vi "MGCC_DataLog.vi"(0 "Start 2":bool=TRUE, 2 "Start":bool=TRUE) -> ()   [LabVIEW 2016]
uses:
  <vilib>/Utility/file.llb/Write Delimited Spreadsheet (DBL).vi
panel:
  in  "Start 3":bool=TRUE
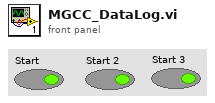
[diagram p1: front panel]
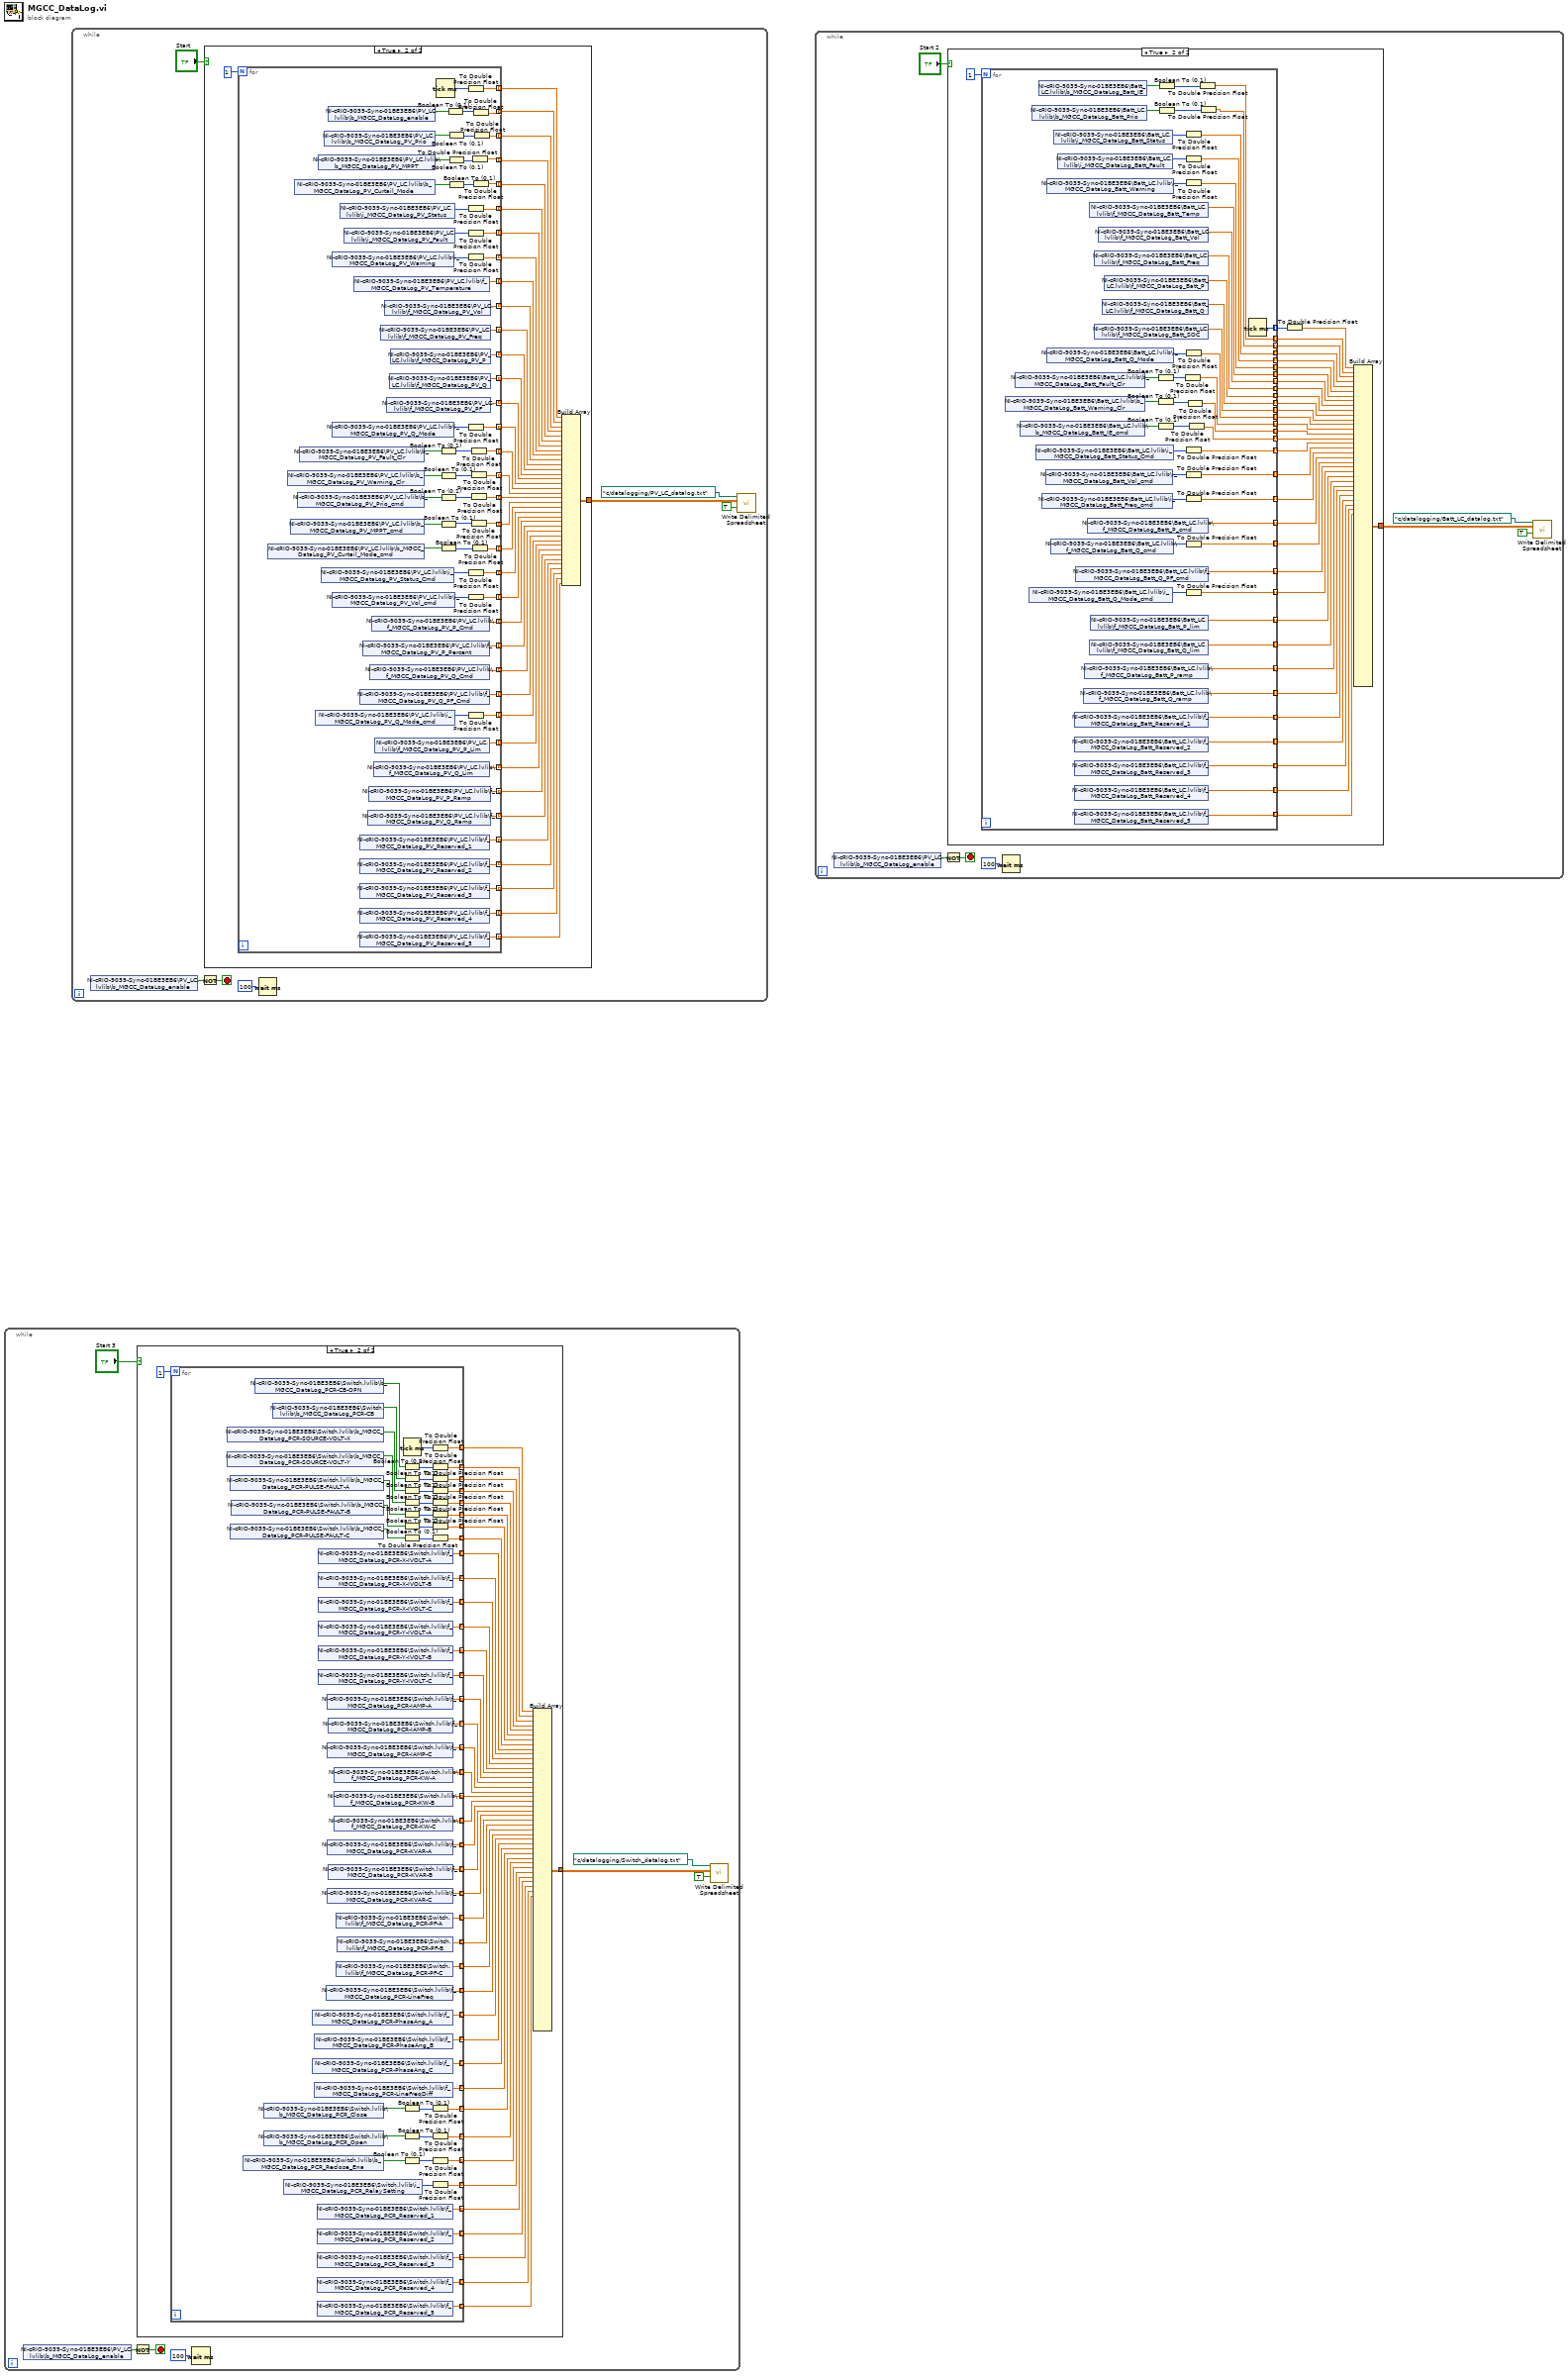
[diagram p0: block diagram]
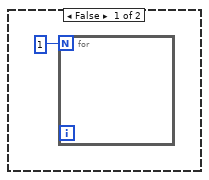
[diagram p2: hidden frame]
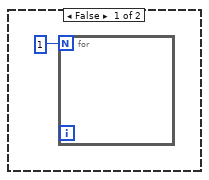
[diagram p3: hidden frame]
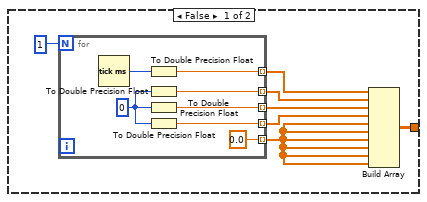
[diagram p4: hidden frame]
diagram:
  n1 = while {
    stop <- w2 stop-if-true
    n2 = shared-variable "NI-cRIO-9039-Sync-01BE3EB6\\PV_LC.lvlib\\b_MGCC_DataLog_enable"() -> (w3:bool)  [unwired: 1 in, 1 out]
    n3 = Not(x=w3) -> (.not. x?=w2:bool)
    n4 = case shown="True" "Start 3" {
      tunnel: [_ w49] -> w7
      frame False {
        n5 = for {
          N: 1 -> [_]
        }
      }
      frame True {
        n6 = for {
          N: 1 -> [_]
          tunnel: [w104] -> w48 mode=indexing
          tunnel: [w101] -> w47 mode=indexing
          tunnel: [w102] -> w46 mode=indexing
          tunnel: [w94] -> w45 mode=indexing
          tunnel: [w93] -> w44 mode=indexing
          tunnel: [w92] -> w43 mode=indexing
          tunnel: [w91] -> w42 mode=indexing
          tunnel: [w90] -> w41 mode=indexing
          tunnel: [w89] -> w40 mode=indexing
          tunnel: [w88] -> w39 mode=indexing
          tunnel: [w87] -> w38 mode=indexing
          tunnel: [w86] -> w37 mode=indexing
          tunnel: [w85] -> w36 mode=indexing
          tunnel: [w84] -> w35 mode=indexing
          tunnel: [w83] -> w34 mode=indexing
          tunnel: [w82] -> w33 mode=indexing
          tunnel: [w81] -> w32 mode=indexing
          tunnel: [w80] -> w31 mode=indexing
          tunnel: [w79] -> w30 mode=indexing
          tunnel: [w78] -> w29 mode=indexing
          tunnel: [w77] -> w28 mode=indexing
          tunnel: [w76] -> w27 mode=indexing
          tunnel: [w75] -> w26 mode=indexing
          tunnel: [w74] -> w25 mode=indexing
          tunnel: [w73] -> w24 mode=indexing
          tunnel: [w72] -> w23 mode=indexing
          tunnel: [w71] -> w22 mode=indexing
          tunnel: [w70] -> w21 mode=indexing
          tunnel: [w69] -> w20 mode=indexing
          tunnel: [w68] -> w19 mode=indexing
          tunnel: [w67] -> w18 mode=indexing
          tunnel: [w59] -> w17 mode=indexing
          tunnel: [w58] -> w16 mode=indexing
          tunnel: [w57] -> w15 mode=indexing
          tunnel: [w56] -> w14 mode=indexing
          tunnel: [w55] -> w13 mode=indexing
          tunnel: [w54] -> w12 mode=indexing
          tunnel: [w53] -> w11 mode=indexing
          tunnel: [w52] -> w10 mode=indexing
          tunnel: [w51] -> w9 mode=indexing
          n7 = shared-variable "NI-cRIO-9039-Sync-01BE3EB6\\Switch.lvlib\\b_MGCC_DataLog_PCR-SOURCE-VOLT-X"() -> (w110:bool)  [unwired: 1 in, 1 out]
          n8 = shared-variable "NI-cRIO-9039-Sync-01BE3EB6\\Switch.lvlib\\b_MGCC_DataLog_PCR-SOURCE-VOLT-Y"() -> (w109:bool)  [unwired: 1 in, 1 out]
          n9 = shared-variable "NI-cRIO-9039-Sync-01BE3EB6\\Switch.lvlib\\b_MGCC_DataLog_PCR-PULSE-FAULT-A"() -> (w108:bool)  [unwired: 1 in, 1 out]
          n10 = shared-variable "NI-cRIO-9039-Sync-01BE3EB6\\Switch.lvlib\\b_MGCC_DataLog_PCR-PULSE-FAULT-C"() -> (w106:bool)  [unwired: 1 in, 1 out]
          n11 = shared-variable "NI-cRIO-9039-Sync-01BE3EB6\\Switch.lvlib\\b_MGCC_DataLog_PCR-PULSE-FAULT-B"() -> (w107:bool)  [unwired: 1 in, 1 out]
          n12 = shared-variable "NI-cRIO-9039-Sync-01BE3EB6\\Switch.lvlib\\b_MGCC_DataLog_PCR_Reclose_Ena"() -> (w62:bool)  [unwired: 1 in, 1 out]
          n13 = shared-variable "NI-cRIO-9039-Sync-01BE3EB6\\Switch.lvlib\\b_MGCC_DataLog_PCR-CB-OPN"() -> (w112:bool)  [unwired: 1 in, 1 out]
          n14 = shared-variable "NI-cRIO-9039-Sync-01BE3EB6\\Switch.lvlib\\b_MGCC_DataLog_PCR_Close"() -> (w66:bool)  [unwired: 1 in, 1 out]
          n15 = shared-variable "NI-cRIO-9039-Sync-01BE3EB6\\Switch.lvlib\\b_MGCC_DataLog_PCR_Open"() -> (w64:bool)  [unwired: 1 in, 1 out]
          n16 = shared-variable "NI-cRIO-9039-Sync-01BE3EB6\\Switch.lvlib\\b_MGCC_DataLog_PCR-CB"() -> (w111:bool)  [unwired: 1 in, 1 out]
          n17 = shared-variable "NI-cRIO-9039-Sync-01BE3EB6\\Switch.lvlib\\i_MGCC_DataLog_PCR_RelaySetting"() -> (w60:i16)  [unwired: 1 in, 1 out]
          n18 = shared-variable "NI-cRIO-9039-Sync-01BE3EB6\\Switch.lvlib\\f_MGCC_DataLog_PCR-PhaseAng_A"() -> (w70:dbl)  [unwired: 1 in, 1 out]
          n19 = shared-variable "NI-cRIO-9039-Sync-01BE3EB6\\Switch.lvlib\\f_MGCC_DataLog_PCR-PhaseAng_C"() -> (w67:dbl)  [unwired: 1 in, 1 out]
          n20 = shared-variable "NI-cRIO-9039-Sync-01BE3EB6\\Switch.lvlib\\f_MGCC_DataLog_PCR-PhaseAng_B"() -> (w69:dbl)  [unwired: 1 in, 1 out]
          n21 = shared-variable "NI-cRIO-9039-Sync-01BE3EB6\\Switch.lvlib\\f_MGCC_DataLog_PCR-LineFreqDiff"() -> (w68:dbl)  [unwired: 1 in, 1 out]
          n22 = shared-variable "NI-cRIO-9039-Sync-01BE3EB6\\Switch.lvlib\\f_MGCC_DataLog_PCR_Reserved_1"() -> (w55:dbl)  [unwired: 1 in, 1 out]
          n23 = shared-variable "NI-cRIO-9039-Sync-01BE3EB6\\Switch.lvlib\\f_MGCC_DataLog_PCR_Reserved_2"() -> (w54:dbl)  [unwired: 1 in, 1 out]
          n24 = shared-variable "NI-cRIO-9039-Sync-01BE3EB6\\Switch.lvlib\\f_MGCC_DataLog_PCR_Reserved_3"() -> (w53:dbl)  [unwired: 1 in, 1 out]
          n25 = shared-variable "NI-cRIO-9039-Sync-01BE3EB6\\Switch.lvlib\\f_MGCC_DataLog_PCR_Reserved_4"() -> (w51:dbl)  [unwired: 1 in, 1 out]
          n26 = shared-variable "NI-cRIO-9039-Sync-01BE3EB6\\Switch.lvlib\\f_MGCC_DataLog_PCR_Reserved_5"() -> (w52:dbl)  [unwired: 1 in, 1 out]
          n27 = shared-variable "NI-cRIO-9039-Sync-01BE3EB6\\Switch.lvlib\\f_MGCC_DataLog_PCR-X-IVOLT-A"() -> (w89:dbl)  [unwired: 1 in, 1 out]
          n28 = shared-variable "NI-cRIO-9039-Sync-01BE3EB6\\Switch.lvlib\\f_MGCC_DataLog_PCR-X-IVOLT-B"() -> (w88:dbl)  [unwired: 1 in, 1 out]
          n29 = shared-variable "NI-cRIO-9039-Sync-01BE3EB6\\Switch.lvlib\\f_MGCC_DataLog_PCR-X-IVOLT-C"() -> (w87:dbl)  [unwired: 1 in, 1 out]
          n30 = shared-variable "NI-cRIO-9039-Sync-01BE3EB6\\Switch.lvlib\\f_MGCC_DataLog_PCR-Y-IVOLT-A"() -> (w86:dbl)  [unwired: 1 in, 1 out]
          n31 = shared-variable "NI-cRIO-9039-Sync-01BE3EB6\\Switch.lvlib\\f_MGCC_DataLog_PCR-Y-IVOLT-B"() -> (w85:dbl)  [unwired: 1 in, 1 out]
          n32 = shared-variable "NI-cRIO-9039-Sync-01BE3EB6\\Switch.lvlib\\f_MGCC_DataLog_PCR-Y-IVOLT-C"() -> (w84:dbl)  [unwired: 1 in, 1 out]
          n33 = shared-variable "NI-cRIO-9039-Sync-01BE3EB6\\Switch.lvlib\\f_MGCC_DataLog_PCR-LineFreq"() -> (w71:dbl)  [unwired: 1 in, 1 out]
          n34 = shared-variable "NI-cRIO-9039-Sync-01BE3EB6\\Switch.lvlib\\f_MGCC_DataLog_PCR-IAMP-A"() -> (w83:dbl)  [unwired: 1 in, 1 out]
          n35 = shared-variable "NI-cRIO-9039-Sync-01BE3EB6\\Switch.lvlib\\f_MGCC_DataLog_PCR-IAMP-C"() -> (w81:dbl)  [unwired: 1 in, 1 out]
          n36 = shared-variable "NI-cRIO-9039-Sync-01BE3EB6\\Switch.lvlib\\f_MGCC_DataLog_PCR-KVAR-A"() -> (w77:dbl)  [unwired: 1 in, 1 out]
          n37 = shared-variable "NI-cRIO-9039-Sync-01BE3EB6\\Switch.lvlib\\f_MGCC_DataLog_PCR-KVAR-C"() -> (w75:dbl)  [unwired: 1 in, 1 out]
          n38 = shared-variable "NI-cRIO-9039-Sync-01BE3EB6\\Switch.lvlib\\f_MGCC_DataLog_PCR-IAMP-B"() -> (w82:dbl)  [unwired: 1 in, 1 out]
          n39 = shared-variable "NI-cRIO-9039-Sync-01BE3EB6\\Switch.lvlib\\f_MGCC_DataLog_PCR-KVAR-B"() -> (w76:dbl)  [unwired: 1 in, 1 out]
          n40 = shared-variable "NI-cRIO-9039-Sync-01BE3EB6\\Switch.lvlib\\f_MGCC_DataLog_PCR-KW-A"() -> (w80:dbl)  [unwired: 1 in, 1 out]
          n41 = shared-variable "NI-cRIO-9039-Sync-01BE3EB6\\Switch.lvlib\\f_MGCC_DataLog_PCR-KW-B"() -> (w79:dbl)  [unwired: 1 in, 1 out]
          n42 = shared-variable "NI-cRIO-9039-Sync-01BE3EB6\\Switch.lvlib\\f_MGCC_DataLog_PCR-KW-C"() -> (w78:dbl)  [unwired: 1 in, 1 out]
          n43 = shared-variable "NI-cRIO-9039-Sync-01BE3EB6\\Switch.lvlib\\f_MGCC_DataLog_PCR-PF-A"() -> (w74:dbl)  [unwired: 1 in, 1 out]
          n44 = shared-variable "NI-cRIO-9039-Sync-01BE3EB6\\Switch.lvlib\\f_MGCC_DataLog_PCR-PF-C"() -> (w72:dbl)  [unwired: 1 in, 1 out]
          n45 = shared-variable "NI-cRIO-9039-Sync-01BE3EB6\\Switch.lvlib\\f_MGCC_DataLog_PCR-PF-B"() -> (w73:dbl)  [unwired: 1 in, 1 out]
          n46 = Boolean To (0,1)(Boolean=w112) -> (0, 1=w100:i16)
          n47 = Boolean To (0,1)(Boolean=w111) -> (0, 1=w103:i16)
          n48 = Boolean To (0,1)(Boolean=w110) -> (0, 1=w95:i16)
          n49 = Boolean To (0,1)(Boolean=w109) -> (0, 1=w96:i16)
          n50 = Boolean To (0,1)(Boolean=w108) -> (0, 1=w97:i16)
          n51 = Boolean To (0,1)(Boolean=w107) -> (0, 1=w98:i16)
          n52 = Boolean To (0,1)(Boolean=w106) -> (0, 1=w99:i16)
          n53 = Boolean To (0,1)(Boolean=w66) -> (0, 1=w65:i16)
          n54 = Boolean To (0,1)(Boolean=w64) -> (0, 1=w63:i16)
          n55 = Boolean To (0,1)(Boolean=w62) -> (0, 1=w61:i16)
          n56 = Tick Count (ms)() -> (millisecond timer value=w105:u32)
          n57 = To Double Precision Float(number=w105) -> (double precision float=w104:dbl)
          n58 = To Double Precision Float(number=w100) -> (double precision float=w101:dbl)
          n59 = To Double Precision Float(number=w103) -> (double precision float=w102:dbl)
          n60 = To Double Precision Float(number=w95) -> (double precision float=w94:dbl)
          n61 = To Double Precision Float(number=w96) -> (double precision float=w93:dbl)
          n62 = To Double Precision Float(number=w97) -> (double precision float=w92:dbl)
          n63 = To Double Precision Float(number=w98) -> (double precision float=w91:dbl)
          n64 = To Double Precision Float(number=w99) -> (double precision float=w90:dbl)
          n65 = To Double Precision Float(number=w65) -> (double precision float=w59:dbl)
          n66 = To Double Precision Float(number=w63) -> (double precision float=w58:dbl)
          n67 = To Double Precision Float(number=w61) -> (double precision float=w57:dbl)
          n68 = To Double Precision Float(number=w60) -> (double precision float=w56:dbl)
        }
        n69 = Build Array(w48, w47, w46, w45, w44, w43, w42, w41, w40, w39, w38, w37, w36, w35, w34, w33, w32, w31, w30, w29, w28, w27, w26, w25, w24, w23, w22, w21, w20, w18, w19, w17, w16, w15, w14, w13, w12, w11, w9, w10) -> (w49:dbl[][])  [unwired: 28 in]
      }
    }
    n70 = Wait (ms)(milliseconds to wait=u32 100) -> ()  [unwired: 1 out]
    n71 = call-poly <vilib>:"Write Delimited Spreadsheet.vi"("file path (dialog if empty)"=path "c:/datalogging/Switch_datalog.txt", "2D data"=w7, "append to file? (new file:F)"=TRUE) -> ()  [unwired: 11 in, 2 out]
  }
  n72 = while {
    stop <- w113 stop-if-true
    n73 = shared-variable "NI-cRIO-9039-Sync-01BE3EB6\\PV_LC.lvlib\\b_MGCC_DataLog_enable"() -> (w114:bool)  [unwired: 1 in, 1 out]
    n74 = Not(x=w114) -> (.not. x?=w113:bool)
    n75 = case shown="True" "Start" {
      tunnel: [w121 w167] -> w116
      frame False {
        n76 = for {
          N: 1 -> [_]
          tunnel: [w133] -> w126 mode=indexing
          tunnel: [w131] -> w125 mode=indexing
          tunnel: [w130] -> w124 mode=indexing
          tunnel: [0.0] -> w123 mode=indexing
          tunnel: [w128] -> w122 mode=indexing
          w132 = 0
          n77 = Tick Count (ms)() -> (millisecond timer value=w127:u32)
          n78 = To Double Precision Float(number=w127) -> (double precision float=w128:dbl)
          n79 = To Double Precision Float(number=w132) -> (double precision float=w133:dbl)
          n80 = To Double Precision Float(number=w132) -> (double precision float=w131:dbl)
          n81 = To Double Precision Float(number=w132) -> (double precision float=w130:dbl)
        }
        n82 = Build Array(w122, w126, w125, w124, w123, w123, w123, w123, w123, w123) -> (w121:dbl[][])
      }
      frame True {
        n83 = for {
          N: 1 -> [_]
          tunnel: [w182] -> w171 mode=indexing
          tunnel: [w184] -> w170 mode=indexing
          tunnel: [w186] -> w169 mode=indexing
          tunnel: [w231] -> w168 mode=indexing
          tunnel: [w188] -> w165 mode=indexing
          tunnel: [w224] -> w164 mode=indexing
          tunnel: [w223] -> w163 mode=indexing
          tunnel: [w222] -> w162 mode=indexing
          tunnel: [w221] -> w161 mode=indexing
          tunnel: [w220] -> w160 mode=indexing
          tunnel: [w219] -> w159 mode=indexing
          tunnel: [w218] -> w158 mode=indexing
          tunnel: [w217] -> w157 mode=indexing
          tunnel: [w216] -> w156 mode=indexing
          tunnel: [w214] -> w155 mode=indexing
          tunnel: [w179] -> w154 mode=indexing
          tunnel: [w180] -> w153 mode=indexing
          tunnel: [w181] -> w152 mode=indexing
          tunnel: [w178] -> w151 mode=indexing
          tunnel: [w177] -> w150 mode=indexing
          tunnel: [w206] -> w149 mode=indexing
          tunnel: [w205] -> w148 mode=indexing
          tunnel: [w204] -> w147 mode=indexing
          tunnel: [w203] -> w146 mode=indexing
          tunnel: [w202] -> w145 mode=indexing
          tunnel: [w201] -> w144 mode=indexing
          tunnel: [w199] -> w143 mode=indexing
          tunnel: [w198] -> w142 mode=indexing
          tunnel: [w197] -> w141 mode=indexing
          tunnel: [w196] -> w140 mode=indexing
          tunnel: [w195] -> w139 mode=indexing
          tunnel: [w194] -> w138 mode=indexing
          tunnel: [w193] -> w137 mode=indexing
          tunnel: [w192] -> w136 mode=indexing
          tunnel: [w191] -> w135 mode=indexing
          tunnel: [w190] -> w134 mode=indexing
          n84 = shared-variable "NI-cRIO-9039-Sync-01BE3EB6\\PV_LC.lvlib\\b_MGCC_DataLog_PV_Curtail_Mode_cmd"() -> (w209:bool)  [unwired: 1 in, 1 out]
          n85 = shared-variable "NI-cRIO-9039-Sync-01BE3EB6\\PV_LC.lvlib\\b_MGCC_DataLog_PV_Warning_Clr"() -> (w212:bool)  [unwired: 1 in, 1 out]
          n86 = shared-variable "NI-cRIO-9039-Sync-01BE3EB6\\PV_LC.lvlib\\b_MGCC_DataLog_PV_MPPT_cmd"() -> (w210:bool)  [unwired: 1 in, 1 out]
          n87 = shared-variable "NI-cRIO-9039-Sync-01BE3EB6\\PV_LC.lvlib\\b_MGCC_DataLog_PV_Curtail_Mode"() -> (w226:bool)  [unwired: 1 in, 1 out]
          n88 = shared-variable "NI-cRIO-9039-Sync-01BE3EB6\\PV_LC.lvlib\\b_MGCC_DataLog_PV_Prio_cmd"() -> (w211:bool)  [unwired: 1 in, 1 out]
          n89 = shared-variable "NI-cRIO-9039-Sync-01BE3EB6\\PV_LC.lvlib\\b_MGCC_DataLog_PV_Fault_Clr"() -> (w213:bool)  [unwired: 1 in, 1 out]
          n90 = shared-variable "NI-cRIO-9039-Sync-01BE3EB6\\PV_LC.lvlib\\i_MGCC_DataLog_PV_Q_Mode_cmd"() -> (w200:i16)  [unwired: 1 in, 1 out]
          n91 = shared-variable "NI-cRIO-9039-Sync-01BE3EB6\\PV_LC.lvlib\\b_MGCC_DataLog_PV_MPPT"() -> (w227:bool)  [unwired: 1 in, 1 out]
          n92 = shared-variable "NI-cRIO-9039-Sync-01BE3EB6\\PV_LC.lvlib\\i_MGCC_DataLog_PV_Status_Cmd"() -> (w207:i16)  [unwired: 1 in, 1 out]
          n93 = shared-variable "NI-cRIO-9039-Sync-01BE3EB6\\PV_LC.lvlib\\b_MGCC_DataLog_PV_Prio"() -> (w228:bool)  [unwired: 1 in, 1 out]
          n94 = shared-variable "NI-cRIO-9039-Sync-01BE3EB6\\PV_LC.lvlib\\b_MGCC_DataLog_enable"() -> (w229:bool)  [unwired: 1 in, 1 out]
          n95 = shared-variable "NI-cRIO-9039-Sync-01BE3EB6\\PV_LC.lvlib\\i_MGCC_DataLog_PV_Warning"() -> (w232:i16)  [unwired: 1 in, 1 out]
          n96 = shared-variable "NI-cRIO-9039-Sync-01BE3EB6\\PV_LC.lvlib\\i_MGCC_DataLog_PV_Q_Mode"() -> (w215:i16)  [unwired: 1 in, 1 out]
          n97 = shared-variable "NI-cRIO-9039-Sync-01BE3EB6\\PV_LC.lvlib\\i_MGCC_DataLog_PV_Vol_cmd"() -> (w208:i16)  [unwired: 1 in, 1 out]
          n98 = shared-variable "NI-cRIO-9039-Sync-01BE3EB6\\PV_LC.lvlib\\i_MGCC_DataLog_PV_Status"() -> (w225:i16)  [unwired: 1 in, 1 out]
          n99 = shared-variable "NI-cRIO-9039-Sync-01BE3EB6\\PV_LC.lvlib\\i_MGCC_DataLog_PV_Fault"() -> (w233:i16)  [unwired: 1 in, 1 out]
          n100 = shared-variable "NI-cRIO-9039-Sync-01BE3EB6\\PV_LC.lvlib\\f_MGCC_DataLog_PV_Temperature"() -> (w221:dbl)  [unwired: 1 in, 1 out]
          n101 = shared-variable "NI-cRIO-9039-Sync-01BE3EB6\\PV_LC.lvlib\\f_MGCC_DataLog_PV_Q_PF_Cmd"() -> (w201:dbl)  [unwired: 1 in, 1 out]
          n102 = shared-variable "NI-cRIO-9039-Sync-01BE3EB6\\PV_LC.lvlib\\f_MGCC_DataLog_PV_Reserved_1"() -> (w194:dbl)  [unwired: 1 in, 1 out]
          n103 = shared-variable "NI-cRIO-9039-Sync-01BE3EB6\\PV_LC.lvlib\\f_MGCC_DataLog_PV_Reserved_2"() -> (w193:dbl)  [unwired: 1 in, 1 out]
          n104 = shared-variable "NI-cRIO-9039-Sync-01BE3EB6\\PV_LC.lvlib\\f_MGCC_DataLog_PV_Reserved_3"() -> (w192:dbl)  [unwired: 1 in, 1 out]
          n105 = shared-variable "NI-cRIO-9039-Sync-01BE3EB6\\PV_LC.lvlib\\f_MGCC_DataLog_PV_Reserved_4"() -> (w191:dbl)  [unwired: 1 in, 1 out]
          n106 = shared-variable "NI-cRIO-9039-Sync-01BE3EB6\\PV_LC.lvlib\\f_MGCC_DataLog_PV_Reserved_5"() -> (w190:dbl)  [unwired: 1 in, 1 out]
          n107 = shared-variable "NI-cRIO-9039-Sync-01BE3EB6\\PV_LC.lvlib\\f_MGCC_DataLog_PV_P_Percent"() -> (w203:dbl)  [unwired: 1 in, 1 out]
          n108 = shared-variable "NI-cRIO-9039-Sync-01BE3EB6\\PV_LC.lvlib\\f_MGCC_DataLog_PV_Q_Ramp"() -> (w195:dbl)  [unwired: 1 in, 1 out]
          n109 = shared-variable "NI-cRIO-9039-Sync-01BE3EB6\\PV_LC.lvlib\\f_MGCC_DataLog_PV_P_Ramp"() -> (w196:dbl)  [unwired: 1 in, 1 out]
          n110 = shared-variable "NI-cRIO-9039-Sync-01BE3EB6\\PV_LC.lvlib\\f_MGCC_DataLog_PV_Q_Cmd"() -> (w202:dbl)  [unwired: 1 in, 1 out]
          n111 = shared-variable "NI-cRIO-9039-Sync-01BE3EB6\\PV_LC.lvlib\\f_MGCC_DataLog_PV_P_Cmd"() -> (w204:dbl)  [unwired: 1 in, 1 out]
          n112 = shared-variable "NI-cRIO-9039-Sync-01BE3EB6\\PV_LC.lvlib\\f_MGCC_DataLog_PV_Q_Lim"() -> (w197:dbl)  [unwired: 1 in, 1 out]
          n113 = shared-variable "NI-cRIO-9039-Sync-01BE3EB6\\PV_LC.lvlib\\f_MGCC_DataLog_PV_P_Lim"() -> (w198:dbl)  [unwired: 1 in, 1 out]
          n114 = shared-variable "NI-cRIO-9039-Sync-01BE3EB6\\PV_LC.lvlib\\f_MGCC_DataLog_PV_Freq"() -> (w219:dbl)  [unwired: 1 in, 1 out]
          n115 = shared-variable "NI-cRIO-9039-Sync-01BE3EB6\\PV_LC.lvlib\\f_MGCC_DataLog_PV_Vol"() -> (w220:dbl)  [unwired: 1 in, 1 out]
          n116 = shared-variable "NI-cRIO-9039-Sync-01BE3EB6\\PV_LC.lvlib\\f_MGCC_DataLog_PV_PF"() -> (w216:dbl)  [unwired: 1 in, 1 out]
          n117 = shared-variable "NI-cRIO-9039-Sync-01BE3EB6\\PV_LC.lvlib\\f_MGCC_DataLog_PV_Q"() -> (w217:dbl)  [unwired: 1 in, 1 out]
          n118 = shared-variable "NI-cRIO-9039-Sync-01BE3EB6\\PV_LC.lvlib\\f_MGCC_DataLog_PV_P"() -> (w218:dbl)  [unwired: 1 in, 1 out]
          n119 = Tick Count (ms)() -> (millisecond timer value=w230:u32)
          n120 = Boolean To (0,1)(Boolean=w213) -> (0, 1=w172:i16)
          n121 = Boolean To (0,1)(Boolean=w212) -> (0, 1=w173:i16)
          n122 = Boolean To (0,1)(Boolean=w211) -> (0, 1=w174:i16)
          n123 = Boolean To (0,1)(Boolean=w210) -> (0, 1=w175:i16)
          n124 = Boolean To (0,1)(Boolean=w209) -> (0, 1=w176:i16)
          n125 = Boolean To (0,1)(Boolean=w229) -> (0, 1=w183:i16)
          n126 = Boolean To (0,1)(Boolean=w228) -> (0, 1=w185:i16)
          n127 = Boolean To (0,1)(Boolean=w227) -> (0, 1=w187:i16)
          n128 = Boolean To (0,1)(Boolean=w226) -> (0, 1=w189:i16)
          n129 = To Double Precision Float(number=w230) -> (double precision float=w231:dbl)
          n130 = To Double Precision Float(number=w225) -> (double precision float=w224:dbl)
          n131 = To Double Precision Float(number=w233) -> (double precision float=w223:dbl)
          n132 = To Double Precision Float(number=w232) -> (double precision float=w222:dbl)
          n133 = To Double Precision Float(number=w215) -> (double precision float=w214:dbl)
          n134 = To Double Precision Float(number=w207) -> (double precision float=w206:dbl)
          n135 = To Double Precision Float(number=w208) -> (double precision float=w205:dbl)
          n136 = To Double Precision Float(number=w200) -> (double precision float=w199:dbl)
          n137 = To Double Precision Float(number=w172) -> (double precision float=w179:dbl)
          n138 = To Double Precision Float(number=w175) -> (double precision float=w178:dbl)
          n139 = To Double Precision Float(number=w173) -> (double precision float=w180:dbl)
          n140 = To Double Precision Float(number=w174) -> (double precision float=w181:dbl)
          n141 = To Double Precision Float(number=w187) -> (double precision float=w186:dbl)
          n142 = To Double Precision Float(number=w176) -> (double precision float=w177:dbl)
          n143 = To Double Precision Float(number=w183) -> (double precision float=w182:dbl)
          n144 = To Double Precision Float(number=w189) -> (double precision float=w188:dbl)
          n145 = To Double Precision Float(number=w185) -> (double precision float=w184:dbl)
        }
        n146 = Build Array(w168, w171, w170, w169, w165, w164, w163, w162, w161, w160, w159, w158, w157, w156, w155, w154, w153, w152, w151, w150, w149, w148, w147, w146, w145, w144, w143, w142, w141, w140, w139, w138, w137, w136, w135, w134) -> (w167:dbl[][])
      }
    }
    n147 = Wait (ms)(milliseconds to wait=u32 100) -> ()  [unwired: 1 out]
    n148 = call-poly <vilib>:"Write Delimited Spreadsheet.vi"("file path (dialog if empty)"=path "c:/datalogging/PV_LC_datalog.txt", "2D data"=w116, "append to file? (new file:F)"=TRUE) -> ()  [unwired: 11 in, 2 out]
  }
  n149 = while {
    stop <- w234 stop-if-true
    n150 = shared-variable "NI-cRIO-9039-Sync-01BE3EB6\\PV_LC.lvlib\\b_MGCC_DataLog_enable"() -> (w235:bool)  [unwired: 1 in, 1 out]
    n151 = Not(x=w235) -> (.not. x?=w234:bool)
    n152 = case shown="True" "Start 2" {
      tunnel: [_ w275] -> w239
      frame False {
        n153 = for {
          N: 1 -> [_]
        }
      }
      frame True {
        n154 = for {
          N: 1 -> [_]
          tunnel: [w327] -> w274 mode=indexing
          tunnel: [w278] -> w272 mode=indexing
          tunnel: [w277] -> w271 mode=indexing
          tunnel: [w313] -> w270 mode=indexing
          tunnel: [w312] -> w269 mode=indexing
          tunnel: [w311] -> w268 mode=indexing
          tunnel: [w310] -> w267 mode=indexing
          tunnel: [w309] -> w266 mode=indexing
          tunnel: [w308] -> w265 mode=indexing
          tunnel: [w307] -> w264 mode=indexing
          tunnel: [w306] -> w263 mode=indexing
          tunnel: [w305] -> w262 mode=indexing
          tunnel: [w303] -> w261 mode=indexing
          tunnel: [w285] -> w260 mode=indexing
          tunnel: [w283] -> w259 mode=indexing
          tunnel: [w281] -> w258 mode=indexing
          tunnel: [w302] -> w257 mode=indexing
          tunnel: [w301] -> w256 mode=indexing
          tunnel: [w300] -> w255 mode=indexing
          tunnel: [w299] -> w254 mode=indexing
          tunnel: [w298] -> w253 mode=indexing
          tunnel: [w297] -> w252 mode=indexing
          tunnel: [w296] -> w251 mode=indexing
          tunnel: [w295] -> w250 mode=indexing
          tunnel: [w294] -> w249 mode=indexing
          tunnel: [w293] -> w248 mode=indexing
          tunnel: [w292] -> w247 mode=indexing
          tunnel: [w291] -> w246 mode=indexing
          tunnel: [w290] -> w245 mode=indexing
          tunnel: [w289] -> w244 mode=indexing
          tunnel: [w288] -> w243 mode=indexing
          tunnel: [w287] -> w242 mode=indexing
          n155 = shared-variable "NI-cRIO-9039-Sync-01BE3EB6\\Batt_LC.lvlib\\b_MGCC_DataLog_Batt_Warning_Clr"() -> (w320:bool)  [unwired: 1 in, 1 out]
          n156 = shared-variable "NI-cRIO-9039-Sync-01BE3EB6\\Batt_LC.lvlib\\b_MGCC_DataLog_Batt_Fault_Clr"() -> (w321:bool)  [unwired: 1 in, 1 out]
          n157 = shared-variable "NI-cRIO-9039-Sync-01BE3EB6\\Batt_LC.lvlib\\b_MGCC_DataLog_Batt_IE_cmd"() -> (w319:bool)  [unwired: 1 in, 1 out]
          n158 = shared-variable "NI-cRIO-9039-Sync-01BE3EB6\\Batt_LC.lvlib\\i_MGCC_DataLog_Batt_Q_Mode_cmd"() -> (w318:i16)  [unwired: 1 in, 1 out]
          n159 = shared-variable "NI-cRIO-9039-Sync-01BE3EB6\\Batt_LC.lvlib\\b_MGCC_DataLog_Batt_Prio"() -> (w322:bool)  [unwired: 1 in, 1 out]
          n160 = shared-variable "NI-cRIO-9039-Sync-01BE3EB6\\Batt_LC.lvlib\\i_MGCC_DataLog_Batt_Status_Cmd"() -> (w315:i16)  [unwired: 1 in, 1 out]
          n161 = shared-variable "NI-cRIO-9039-Sync-01BE3EB6\\Batt_LC.lvlib\\b_MGCC_DataLog_Batt_IE"() -> (w323:bool)  [unwired: 1 in, 1 out]
          n162 = shared-variable "NI-cRIO-9039-Sync-01BE3EB6\\Batt_LC.lvlib\\i_MGCC_DataLog_Batt_Freq_cmd"() -> (w314:i16)  [unwired: 1 in, 1 out]
          n163 = shared-variable "NI-cRIO-9039-Sync-01BE3EB6\\Batt_LC.lvlib\\i_MGCC_DataLog_Batt_Vol_cmd"() -> (w316:i16)  [unwired: 1 in, 1 out]
          n164 = shared-variable "NI-cRIO-9039-Sync-01BE3EB6\\Batt_LC.lvlib\\i_MGCC_DataLog_Batt_Warning"() -> (w324:i16)  [unwired: 1 in, 1 out]
          n165 = shared-variable "NI-cRIO-9039-Sync-01BE3EB6\\Batt_LC.lvlib\\i_MGCC_DataLog_Batt_Q_Mode"() -> (w304:i16)  [unwired: 1 in, 1 out]
          n166 = shared-variable "NI-cRIO-9039-Sync-01BE3EB6\\Batt_LC.lvlib\\f_MGCC_DataLog_Batt_Q_cmd"() -> (w317:i16)  [unwired: 1 in, 1 out]
          n167 = shared-variable "NI-cRIO-9039-Sync-01BE3EB6\\Batt_LC.lvlib\\i_MGCC_DataLog_Batt_Status"() -> (w326:i16)  [unwired: 1 in, 1 out]
          n168 = shared-variable "NI-cRIO-9039-Sync-01BE3EB6\\Batt_LC.lvlib\\i_MGCC_DataLog_Batt_Fault"() -> (w325:i16)  [unwired: 1 in, 1 out]
          n169 = shared-variable "NI-cRIO-9039-Sync-01BE3EB6\\Batt_LC.lvlib\\f_MGCC_DataLog_Batt_Reserved_1"() -> (w291:dbl)  [unwired: 1 in, 1 out]
          n170 = shared-variable "NI-cRIO-9039-Sync-01BE3EB6\\Batt_LC.lvlib\\f_MGCC_DataLog_Batt_Reserved_2"() -> (w290:dbl)  [unwired: 1 in, 1 out]
          n171 = shared-variable "NI-cRIO-9039-Sync-01BE3EB6\\Batt_LC.lvlib\\f_MGCC_DataLog_Batt_Reserved_3"() -> (w289:dbl)  [unwired: 1 in, 1 out]
          n172 = shared-variable "NI-cRIO-9039-Sync-01BE3EB6\\Batt_LC.lvlib\\f_MGCC_DataLog_Batt_Reserved_4"() -> (w288:dbl)  [unwired: 1 in, 1 out]
          n173 = shared-variable "NI-cRIO-9039-Sync-01BE3EB6\\Batt_LC.lvlib\\f_MGCC_DataLog_Batt_Reserved_5"() -> (w287:dbl)  [unwired: 1 in, 1 out]
          n174 = shared-variable "NI-cRIO-9039-Sync-01BE3EB6\\Batt_LC.lvlib\\f_MGCC_DataLog_Batt_Q_PF_cmd"() -> (w297:dbl)  [unwired: 1 in, 1 out]
          n175 = shared-variable "NI-cRIO-9039-Sync-01BE3EB6\\Batt_LC.lvlib\\f_MGCC_DataLog_Batt_Q_ramp"() -> (w292:dbl)  [unwired: 1 in, 1 out]
          n176 = shared-variable "NI-cRIO-9039-Sync-01BE3EB6\\Batt_LC.lvlib\\f_MGCC_DataLog_Batt_P_ramp"() -> (w293:dbl)  [unwired: 1 in, 1 out]
          n177 = shared-variable "NI-cRIO-9039-Sync-01BE3EB6\\Batt_LC.lvlib\\f_MGCC_DataLog_Batt_P_cmd"() -> (w299:dbl)  [unwired: 1 in, 1 out]
          n178 = shared-variable "NI-cRIO-9039-Sync-01BE3EB6\\Batt_LC.lvlib\\f_MGCC_DataLog_Batt_Temp"() -> (w310:dbl)  [unwired: 1 in, 1 out]
          n179 = shared-variable "NI-cRIO-9039-Sync-01BE3EB6\\Batt_LC.lvlib\\f_MGCC_DataLog_Batt_Q_lim"() -> (w294:dbl)  [unwired: 1 in, 1 out]
          n180 = shared-variable "NI-cRIO-9039-Sync-01BE3EB6\\Batt_LC.lvlib\\f_MGCC_DataLog_Batt_P_lim"() -> (w295:dbl)  [unwired: 1 in, 1 out]
          n181 = shared-variable "NI-cRIO-9039-Sync-01BE3EB6\\Batt_LC.lvlib\\f_MGCC_DataLog_Batt_Freq"() -> (w308:dbl)  [unwired: 1 in, 1 out]
          n182 = shared-variable "NI-cRIO-9039-Sync-01BE3EB6\\Batt_LC.lvlib\\f_MGCC_DataLog_Batt_SOC"() -> (w305:dbl)  [unwired: 1 in, 1 out]
          n183 = shared-variable "NI-cRIO-9039-Sync-01BE3EB6\\Batt_LC.lvlib\\f_MGCC_DataLog_Batt_Vol"() -> (w309:dbl)  [unwired: 1 in, 1 out]
          n184 = shared-variable "NI-cRIO-9039-Sync-01BE3EB6\\Batt_LC.lvlib\\f_MGCC_DataLog_Batt_Q"() -> (w306:dbl)  [unwired: 1 in, 1 out]
          n185 = shared-variable "NI-cRIO-9039-Sync-01BE3EB6\\Batt_LC.lvlib\\f_MGCC_DataLog_Batt_P"() -> (w307:dbl)  [unwired: 1 in, 1 out]
          n186 = Boolean To (0,1)(Boolean=w321) -> (0, 1=w286:i16)
          n187 = Boolean To (0,1)(Boolean=w320) -> (0, 1=w284:i16)
          n188 = Boolean To (0,1)(Boolean=w319) -> (0, 1=w282:i16)
          n189 = Boolean To (0,1)(Boolean=w323) -> (0, 1=w279:i16)
          n190 = Boolean To (0,1)(Boolean=w322) -> (0, 1=w280:i16)
          n191 = To Double Precision Float(number=w286) -> (double precision float=w285:dbl)
          n192 = To Double Precision Float(number=w326) -> (double precision float=w313:dbl)
          n193 = To Double Precision Float(number=w325) -> (double precision float=w312:dbl)
          n194 = To Double Precision Float(number=w324) -> (double precision float=w311:dbl)
          n195 = To Double Precision Float(number=w304) -> (double precision float=w303:dbl)
          n196 = To Double Precision Float(number=w315) -> (double precision float=w302:dbl)
          n197 = To Double Precision Float(number=w316) -> (double precision float=w301:dbl)
          n198 = To Double Precision Float(number=w314) -> (double precision float=w300:dbl)
          n199 = To Double Precision Float(number=w317) -> (double precision float=w298:dbl)
          n200 = To Double Precision Float(number=w318) -> (double precision float=w296:dbl)
          n201 = To Double Precision Float(number=w284) -> (double precision float=w283:dbl)
          n202 = To Double Precision Float(number=w282) -> (double precision float=w281:dbl)
          n203 = To Double Precision Float(number=w279) -> (double precision float=w278:dbl)
          n204 = To Double Precision Float(number=w280) -> (double precision float=w277:dbl)
          n205 = Tick Count (ms)() -> (millisecond timer value=w327:u32)
        }
        n206 = To Double Precision Float(number=w274) -> (double precision float=w273:dbl[])
        n207 = Build Array(w273, w272, w271, w270, w269, w268, w267, w266, w265, w264, w263, w262, w261, w260, w259, w258, w257, w256, w255, w254, w253, w252, w251, w250, w249, w248, w247, w246, w245, w244, w243, w242) -> (w275:dbl[][])  [unwired: 36 in]
      }
    }
    n208 = Wait (ms)(milliseconds to wait=u32 100) -> ()  [unwired: 1 out]
    n209 = call-poly <vilib>:"Write Delimited Spreadsheet.vi"("file path (dialog if empty)"=path "c:/datalogging/Batt_LC_datalog.txt", "2D data"=w239, "append to file? (new file:F)"=TRUE) -> ()  [unwired: 11 in, 2 out]
  }
